vi "Send Core.vi"(6 "Severity Code (info)":T1=enum."info", 8 "Error In":errorcluster, 9 "Message Content":string, 10 "Message Tag":string, 11 "CS++MessageLogger in":refnum<class "CS++MessageLogger.lvclass">) -> (0 "Error Out":errorcluster, 3 "CS++MessageLogger out":refnum<class "CS++MessageLogger.lvclass">)   [LabVIEW 2014, in "CS++BaseClasses.lvlib" / "CS++MessageLogger.lvclass"]
doc: "Send mesage to message logger."
uses:
  CS++MessageLogger.lvclass
  Libraries/Base/Severity.ctl
  Libraries/Base/CS++Base.lvlib
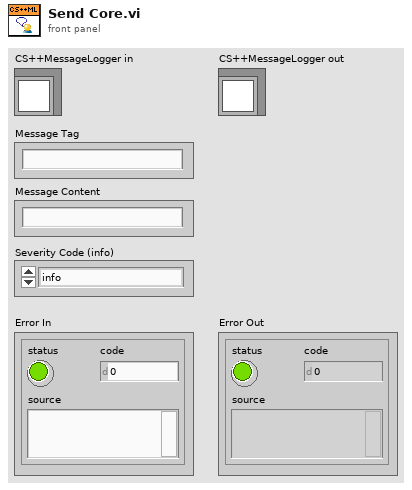
[diagram p1: front panel]
types:
  T1 = typedef "CS++Base.lvlib/Severity.ctl" = enum16{"emergency", "alert", "critical", "error", "warning", "notice", "info", "debug"}
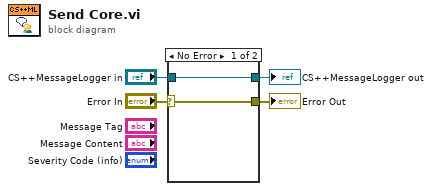
[diagram p0: block diagram]
diagram:
  n1 = case shown="No Error" "Error In" {
    selector: "Error In" -> [w5 w8]
    tunnel: [w5 w8] -> w3
    tunnel: [w6 w7] -> w1
    tunnel: "CS++MessageLogger in" -> [w6 w7]
    frame No Error {
    }
    frame Error {
    }
  }
  "Error Out" <- w3
  "CS++MessageLogger out" <- w1
